vi "Configure I2C Device.vi"(8 "error in (no error)":errorcluster, 10 "I2C Device Configuration":T2, 11 "Device In":T1) -> (0 "error out":errorcluster, 3 "Device out":T1)   [LabVIEW 2016]
uses:
  Type Definitions/I2C Device Configuration.ctl
  <vilib>/ni845x/ni845x.llb/ni845xControl.ctl
  <resource>/objmgr/NI845x.rc
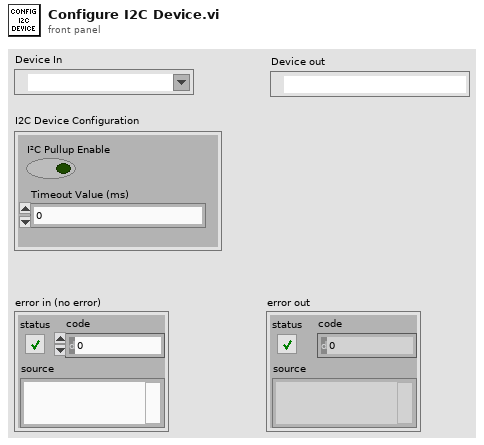
[diagram p1: front panel]
types:
  T1 = typedef "ni845xControl.ctl" = refnum<k21>
  T2 = typedef "I2C Device Configuration.ctl" = cluster{"I²C Pullup Enable":bool, "Timeout Value (ms)":u32}
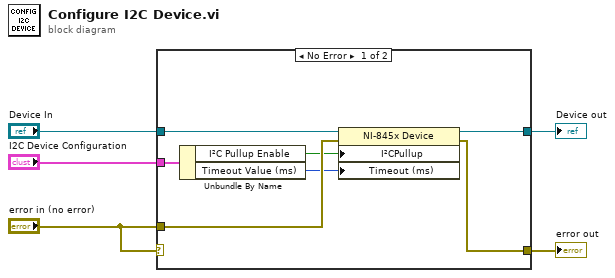
[diagram p0: block diagram]
diagram:
  n1 = case shown="No Error" "error in (no error)" {
    selector: "error in (no error)" -> [_ w14]
    tunnel: "error in (no error)" -> [w12 _]
    tunnel: "I2C Device Configuration" -> [w11 _]
    tunnel: [w8 w14] -> w4
    tunnel: [w7 w13] -> w5
    tunnel: "Device In" -> [w6 w13]
    frame No Error {
      n2 = Unbundle By Name(w11) -> ("I²C Pullup Enable"=w10:bool, "Timeout Value (ms)"=w9:u32)
      n3 = property on="Property Node" class="NI-845x Device"(reference=w6, error in=w12, "I²CPullup"=w10, "Timeout (ms)"=w9) -> (reference out=w7:T1, error out=w8:errorcluster)
    }
    frame Error {
    }
  }
  "error out" <- w4
  "Device out" <- w5
